vi "Modbus_Fetch_Register.vi"(6 "延遲":u32=300, 7 "站號":u8, 8 "error in (no error)":errorcluster, 9 "結束位址":u16, 10 "起始位址":u16, 11 "Modbus Master in":refnum<class "Modbus Master.lvclass">) -> (0 "error out":errorcluster, 2 "register values":u16[](array[numeric]), 3 "Modbus Master out":refnum<class "Modbus Master.lvclass">)   [LabVIEW 2019]
uses:
  <vilib>/NI/Modbus Library/API/Master/Modbus Master.lvclass
  C:/Program Files (x86)/National Instruments/LabVIEW 2019/vi.lib/NI/Modbus Library/API/Modbus API.lvclass
  <vilib>/NI/Modbus Library/API/Modbus API.lvclass/Modbus API.ctl
  <vilib>/NI/Modbus Library/Transmission Data Unit/Transmission Data Unit.lvclass/Transmission Data Unit.ctl
  <vilib>/NI/Modbus Library/Transmission Data Unit/Write Unit ID.vi
  <vilib>/NI/Modbus Library/API/Read Transmission Data Unit.vi
  <vilib>/NI/Modbus Library/API/Write Transmission Data Unit.vi
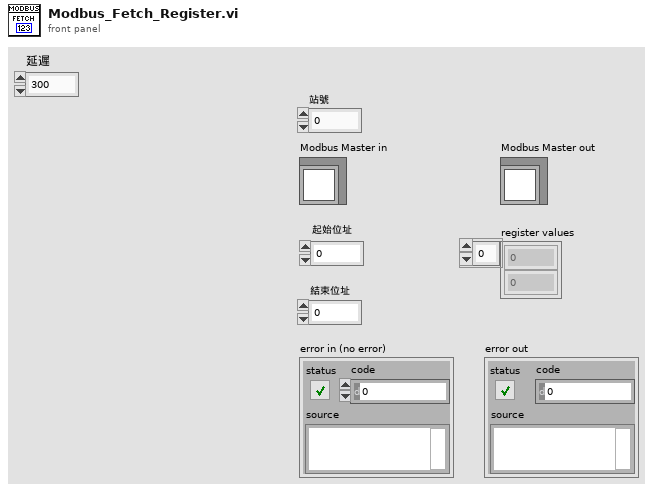
[diagram p1: front panel]
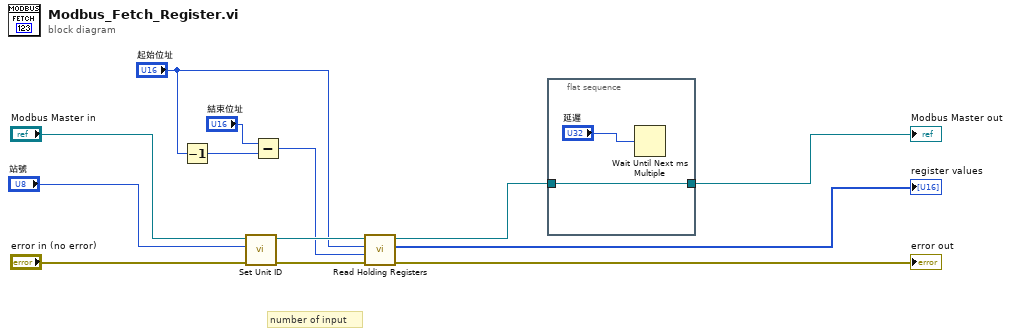
[diagram p0: block diagram]
diagram:
  # "number of input"
  n1 = Decrement(x="起始位址") -> (x-1=w4:u16)
  n2 = call <vilib>:"Set Unit ID.vi"("error in"="error in (no error)", "unit ID"="站號", "Modbus master in"="Modbus Master in") -> ("error out"=w8:errorcluster, "Modbus master out"=w9:refnum<class "Modbus Master.lvclass">)  [unwired: 7 in]
  n3 = Subtract(x="結束位址", y=w4) -> (x-y=w3:u16)
  n4 = call-dynamic "Read Holding Registers.vi"("error in"=w8, "number of inputs"=w3, "starting address"="起始位址", "Modbus master in"=w9) -> ("error out"=→"error out":errorcluster, "register values"=→"register values":u16[], "Modbus master out"=w2:refnum<class "Modbus Master.lvclass">)  [unwired: 5 in]
  n5 = flat-sequence {
    tunnel: w2 -> [w15]
    tunnel: [w15] -> w1
    frame #0 {
      n6 = Wait Until Next ms Multiple(millisecond multiple="延遲") -> ()  [unwired: 1 out]
    }
  }
  "Modbus Master out" <- w1
